vi "lol.vi"(8 "error in":errorcluster) -> (0 "error out":errorcluster, 2 "element":string)   [LabVIEW 2018]
panel:
  out "Image Out":T1(plugin-control)
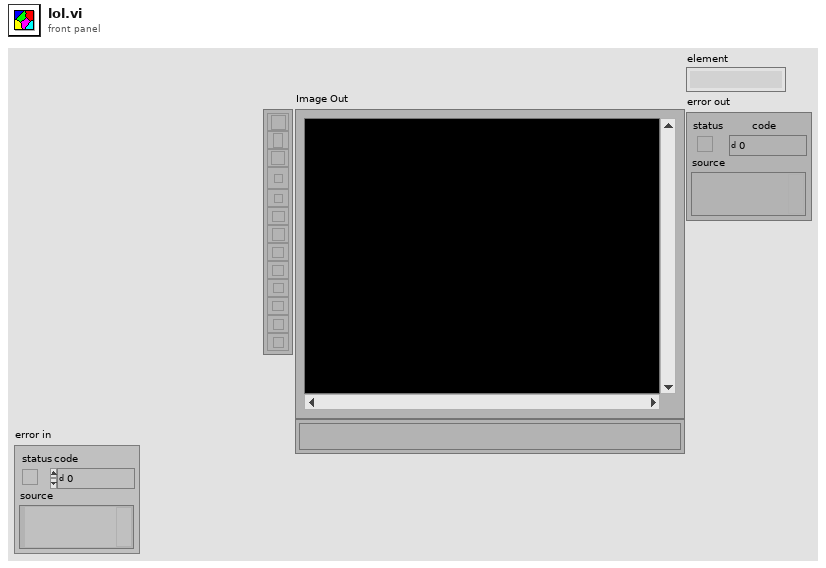
[diagram p1: front panel]
types:
  T1 = typedef "IMAQ Image.ctl" = refnum<image>
  T2 = cluster{"Global Rectangle":i32[], "Contours":cluster{"ID":enum32{"External", "Internal"}, "Type":u32, "Coordinates":i32[]}[]}
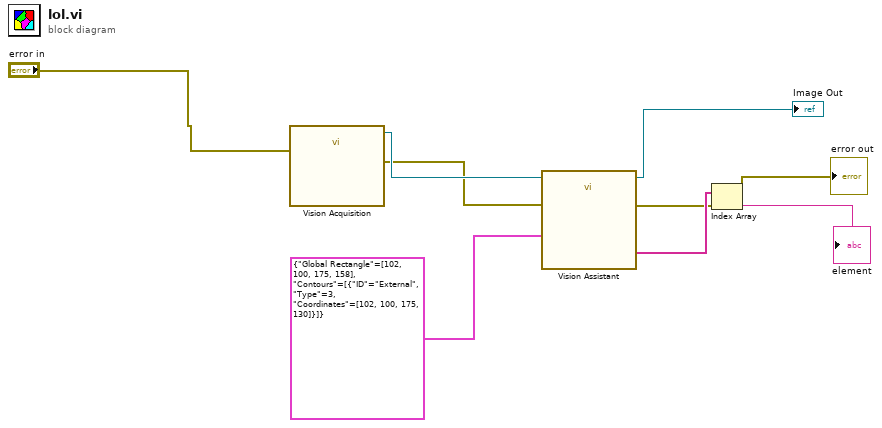
[diagram p0: block diagram]
diagram:
  n1 = call "Vision Acquisition"("error in"="error in") -> ("Image Out"=w7:T1, "error out"=w2:errorcluster)  [unwired: 25 in]
  n2 = call "Vision Assistant"("Image In"=w7, "ROI Descriptor (Color Classification 1)"=T2 {"Global Rectangle"=[102, 100, 175, 158], "Contours"=[{"ID"=enum."External", "Type"=3, "Coordinates"=[102, 100, 175, 130]}]}, "error in"=w2) -> ("Image Out"=→"Image Out":T1, "Classes (Color Classification 1)"=w4:string[], "error out"=→"error out":errorcluster)  [unwired: 22 in]
  n3 = Index Array(array=w4) -> (element=→"element":string)  [unwired: 1 in]
